vi "BKPrecision_PS_Initialize.vi"(6 "Current Limit (0)":dbl=3.0 min=0.0 max=6.0 format="%#.2g", 8 "error in (no error)":errorcluster, 9 "Output Voltage (0)":dbl min=0.0 max=31.0 format="%#.2f", 10 "Maximum Output Voltage (31)":dbl=31.0 min=0.0 max=31.0 format="%#.2f", 11 "VISA resource name":refnum<visa-resource-name>) -> (0 "error out":errorcluster, 3 "VISA resource name out":refnum<visa-resource-name>)   [LabVIEW 2015]
uses:
  <instrlib>/BK Precision 178XB Series/BK Precision 178XB Series.lvlib
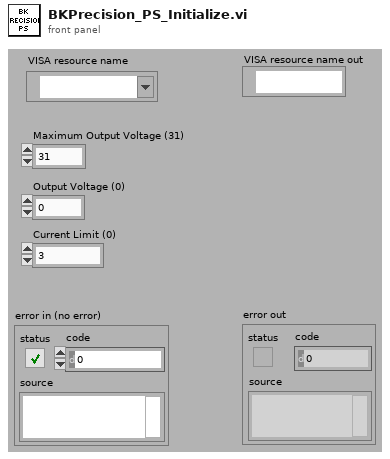
[diagram p1: front panel]
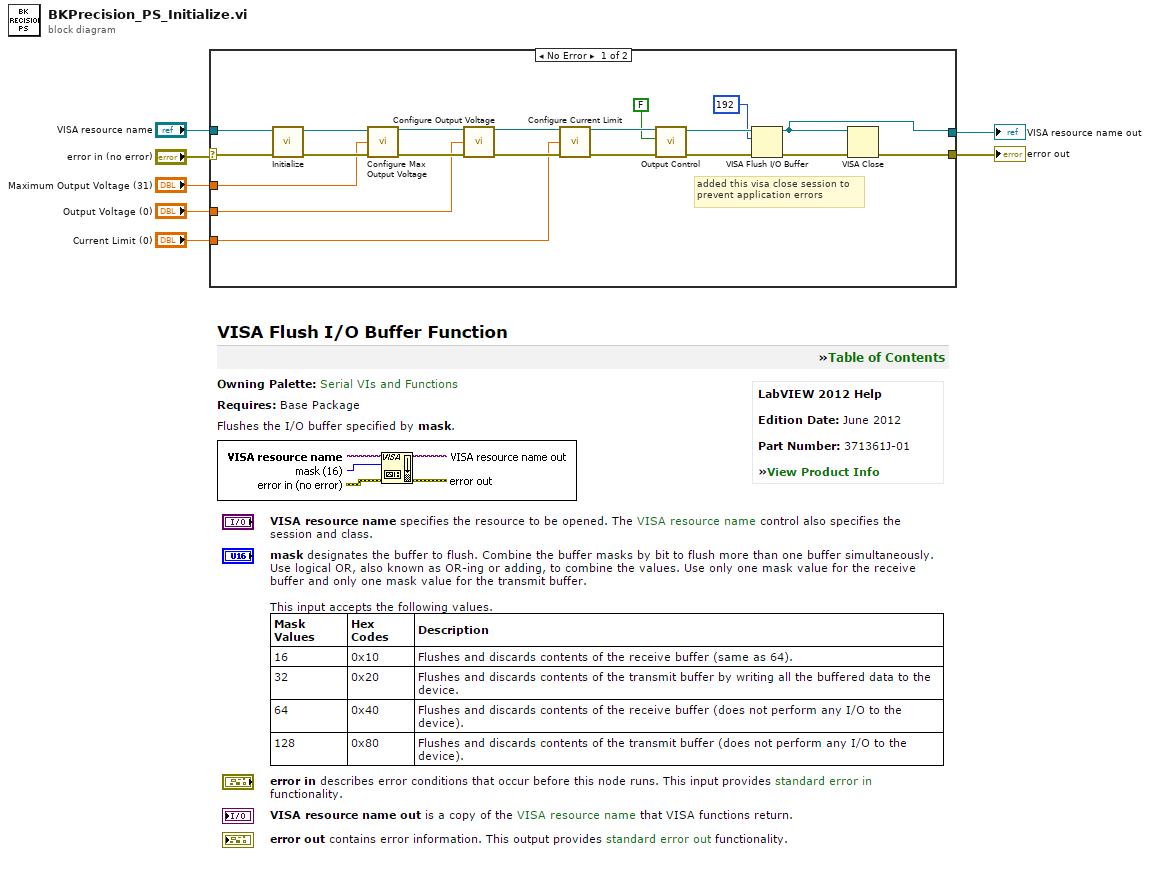
[diagram p0: block diagram]
diagram:
  n1 = case shown="No Error" "error in (no error)" {
    selector: "error in (no error)" -> [w14 w29]
    tunnel: "Maximum Output Voltage (31)" -> [w19 _]
    tunnel: "Output Voltage (0)" -> [w18 _]
    tunnel: "Current Limit (0)" -> [w17 _]
    tunnel: [w10 w29] -> w4
    tunnel: "VISA resource name" -> [w15 w28]
    tunnel: [w9 w28] -> w2
    frame No Error {
      # "added this visa close session to \nprevent application errors"
      n2 = call <instrlib>:"Initialize.vi"("error in (no error)"=w14, "VISA resource name"=w15) -> ("error out"=w26:errorcluster, "VISA resource name out"=w27:refnum<visa-resource-name>)  [unwired: 8 in]
      n3 = call <instrlib>:"Configure Max Output Voltage.vi"("VISA resource name"=w27, "Maximum Output Voltage (18)"=w19, "error in (no error)"=w26) -> ("VISA resource name out"=w25:refnum<visa-resource-name>, "error out"=w22:errorcluster)  [unwired: 11 in]
      n4 = call <instrlib>:"Configure Output Voltage.vi"("VISA resource name"=w25, "Output Voltage (0)"=w18, "error in (no error)"=w22) -> ("VISA resource name out"=w24:refnum<visa-resource-name>, "error out"=w23:errorcluster)  [unwired: 11 in]
      n5 = call <instrlib>:"Configure Current Limit.vi"("VISA resource name"=w24, "Current Limit (0)"=w17, "error in (no error)"=w23) -> ("VISA resource name out"=w21:refnum<visa-resource-name>, "error out"=w20:errorcluster)  [unwired: 11 in]
      n6 = call <instrlib>:"Output Control.vi"("error in (no error)"=w20, "Enable Output Terminals (F: Off)"=FALSE ("off"), "VISA resource name"=w21) -> ("error out"=w11:errorcluster, "VISA resource name out"=w12:refnum<visa-resource-name>)  [unwired: 7 in]
      n7 = VISA Flush I/O Buffer(VISA resource name=w12, mask (16)=u16 192, error in (no error)=w11) -> (VISA resource name out=w9:refnum<visa-resource-name>, error out=w13:errorcluster)
      n8 = VISA Close(VISA resource name=w9, error in (no error)=w13) -> (error out=w10:errorcluster)
    }
    frame Error {
    }
  }
  "error out" <- w4
  "VISA resource name out" <- w2
